vi "Ejemplo de como llamar un modulo.vi"() -> ()   [LabVIEW 2019]
uses:
  Libraries/Plantilla/Plantilla.lvlib
panel:
  out "Status Updated":string
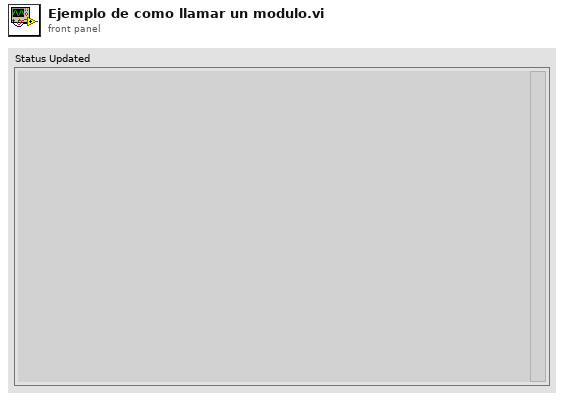
[diagram p1: front panel]
types:
  T1 = typedef "Plantilla.lvlib/Broadcast Events--cluster.ctl" = cluster{"Module Did Init":refnum<user-event>, "Status Updated":refnum<user-event>, "Error Reported":refnum<user-event>, "Module Did Stop":refnum<user-event>, "Update Module Execution Status":refnum<user-event>}
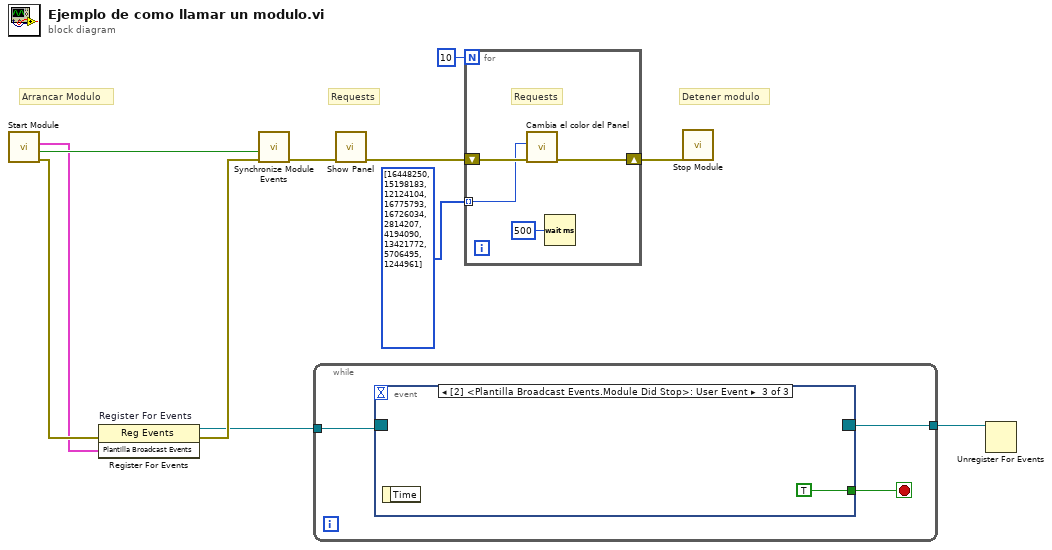
[diagram p0: block diagram]
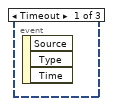
[diagram p2: hidden frame]
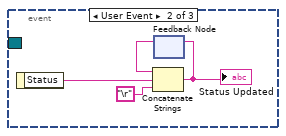
[diagram p3: hidden frame]
diagram:
  # "Requests"
  # "Detener modulo"
  # "Arrancar Modulo"
  n1 = call "Start Module.vi"() -> ("error out"=w5:errorcluster, "Wait for Event Sync?"=w11:bool, "Plantilla Broadcast Events"=w3:T1)  [unwired: 7 in, 2 out]
  n2 = register-events "Register For Events"(error in=w5, w3) -> (reference out=w2:refnum<event-registration>, error out=w4:errorcluster)  [unwired: 1 in]
  n3 = call "Synchronize Module Events.vi"("error in"=w4, "Wait for Event Sync?"=w11) -> ("error out"=w10:errorcluster)  [unwired: 9 in]
  n4 = while {
    tunnel: w2 -> [w14]
    tunnel: [w13] -> w1
    stop <- w12 stop-if-true
    n5 = event shown="[2] <Plantilla Broadcast Events.Module Did Stop>: User Event" {
      selector: w14 -> [_ _ _]
      dyn-events: [_ _ _] -> w13
      timeout: _ -> [_ _ _]
      tunnel: [_ _ TRUE] -> w12
      event Timeout {
        n6 = event-data() -> ()  [unwired: 1 in, 3 out]
      }
      event User Event {
        n7 = event-data() -> ("Status"=w18:string)  [unwired: 1 in]
        n8 = feedback #1() -> (w16:string)  [unwired: 1 in]
        n9 = Concatenate Strings(w16, w18, "\r") -> (w17:string)
        "Status Updated" <- w17
        n10 = feedback-in #1(w17) -> ()
      }
      event User Event {
        n11 = event-data() -> ()  [unwired: 1 in, 1 out]
      }
    }
  }
  n12 = call "Show Panel.vi"("error in"=w10) -> ("error out"=w9:errorcluster)  [unwired: 10 in]
  n13 = for {
    N: 10 -> [_]
    shift-right: [w22] -> w8
    shift-left: w9 -> [w23]
    tunnel: u32[] [16448250, 15198183, 12124104, 16775793, 16726034, 2814207, 4194090, 13421772, 5706495, 1244961] ("Color del Panel") -> [w20] mode=indexing
    # "Requests"
    n14 = call "Cambia el color del Panel.vi"("error in"=w23, "Color del Panel"=w20) -> ("error out"=w22:errorcluster)  [unwired: 9 in]
    n15 = Wait (ms)(milliseconds to wait=u32 500) -> ()  [unwired: 1 out]
  }
  n16 = call "Stop Module.vi"("error in"=w8) -> ()  [unwired: 10 in, 1 out]
  n17 = Unregister For Events(event registration refnum=w1) -> ()  [unwired: 1 in, 1 out]
